vi "macro_Digital_AndMany.vi"   [LabVIEW 2019, in "Trajectory_Library.lvlib"]
uses:
  Trajectory_Library.lvlib
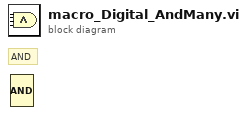
[diagram p0: block diagram]
diagram:
  # "AND"
  n1 = Compound Arithmetic op=AND() -> ()  [unwired: 4 in, 1 out]
